vi "AddResultToListbox.vi"(10 "Results Array in":string[](array[string]), 11 "Lens thickness average":dbl) -> (2 "Formatted results array out":string[](array[string]), 3 "Results Array out":string[](array[string]))   [LabVIEW 2013]
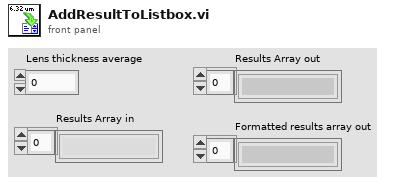
[diagram p1: front panel]
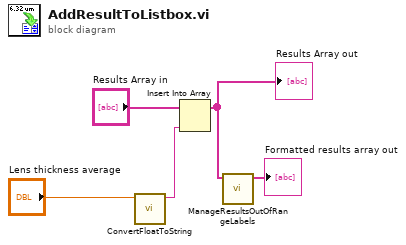
[diagram p0: block diagram]
diagram:
  n1 = call "ConvertFloatToString.vi"("thickness average"="Lens thickness average") -> ("String"=w3:string)  [unwired: 10 in]
  n2 = Insert Into Array(array="Results Array in", new element=w3) -> (w5:string[])  [unwired: 1 in]
  "Results Array out" <- w5
  n3 = call "ManageResultsOutOfRangeLabels.vi"("Input Array 2"=w5) -> ("Input Array 3"=→"Formatted results array out":string[])  [unwired: 10 in]
